vi "HEWH GEA2 Change Mod Sequence.vi"(0 "ComPort":refnum<visa-resource-name>="COM1", 5 "Mode In":T1=enum."StdElectric", 11 "Error In":errorcluster) -> (6 "Mode Set":bool, 15 "Error Out":errorcluster)   [LabVIEW 2009]
uses:
  GEA2/HEWH_Mode.ctl
panel:
  in  "Change Mode Sequence":bool
  in  "Change Mode":bool
  in  "Change Set Point":bool
  in  "Set Point":u8=130
  out "Mode":T1=enum."HighDemand"
  in  "Get Status":bool
  out "Current SetPoint":u8
  in  "OK":bool
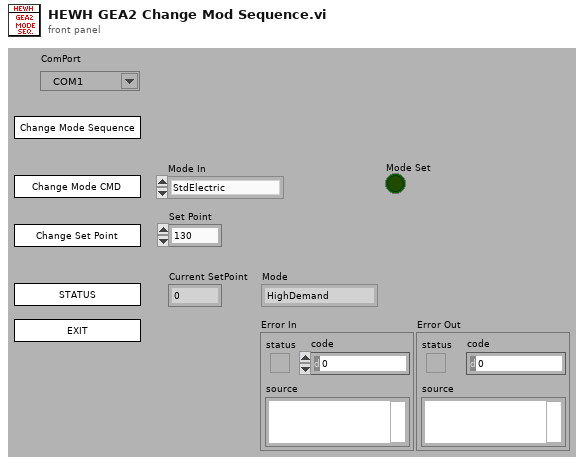
[diagram p1: front panel]
types:
  T1 = typedef "HEWH_Mode.ctl" = enum16{"Hybrid", "StdElectric", "eHeat", "HighDemand", "Unknown"}
  T2 = enum32{"invalid app kind", "Development System", "Run Time System", "Student Edition", "Embedded LabVIEW", "Evaluation", "Custom"}
  T3 = enum32{"Invalid", "Standard", "Closed", "Hidden", "Minimized", "Maximized"}
  T4 = cluster{"Core":cluster{"Current VI Reference":refnum<vi>, "Close Panel on Exit?":bool}, "ComPort":refnum<visa-resource-name>, "Set Point":u8, "Mode In":T1, "Error Status":bool}
  T5 = cluster{"Current VI Reference":refnum<vi>, "Close Panel on Exit?":bool}
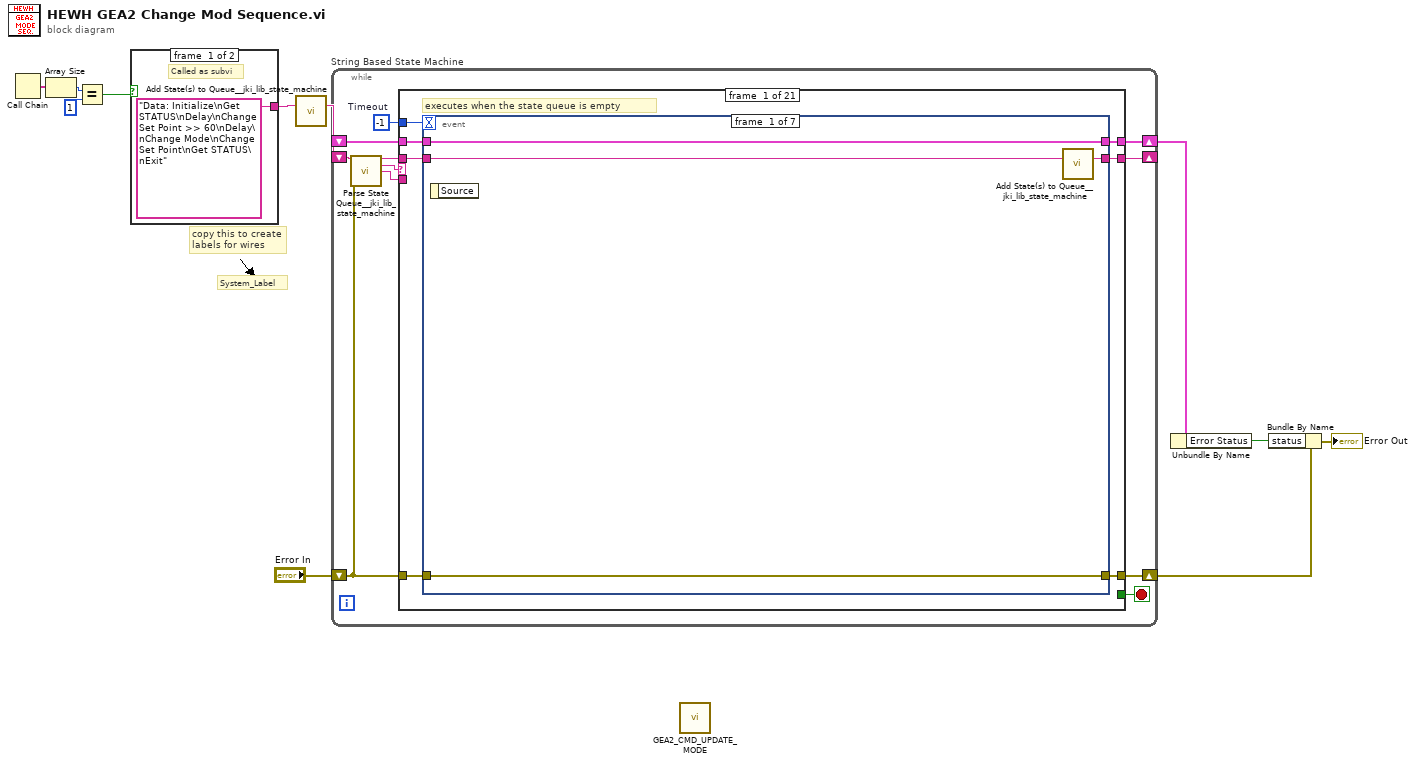
[diagram p0: block diagram]
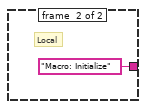
[diagram p2: hidden frame]
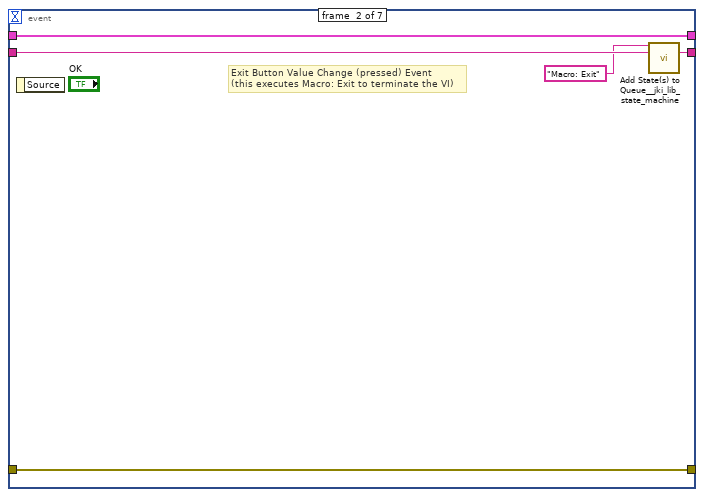
[diagram p3: hidden frame]
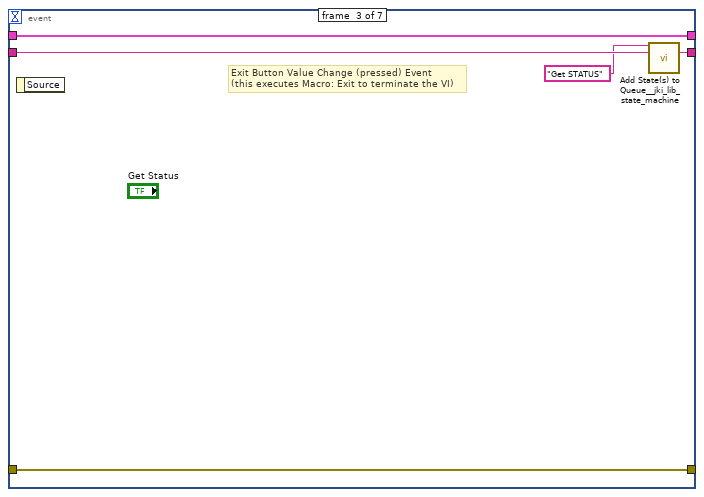
[diagram p4: hidden frame]
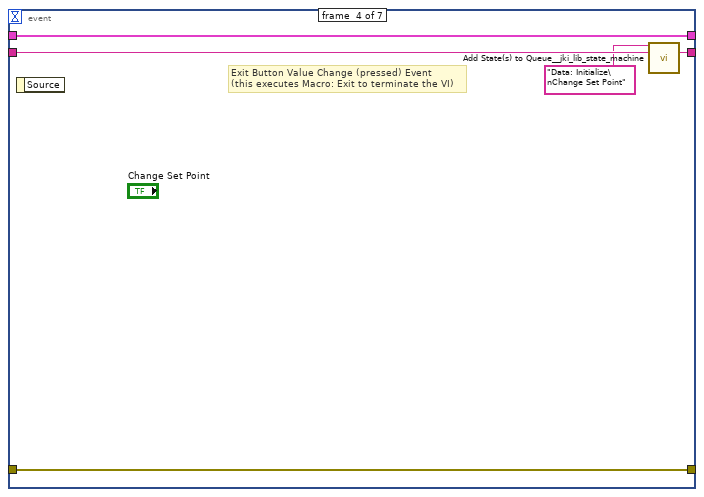
[diagram p5: hidden frame]
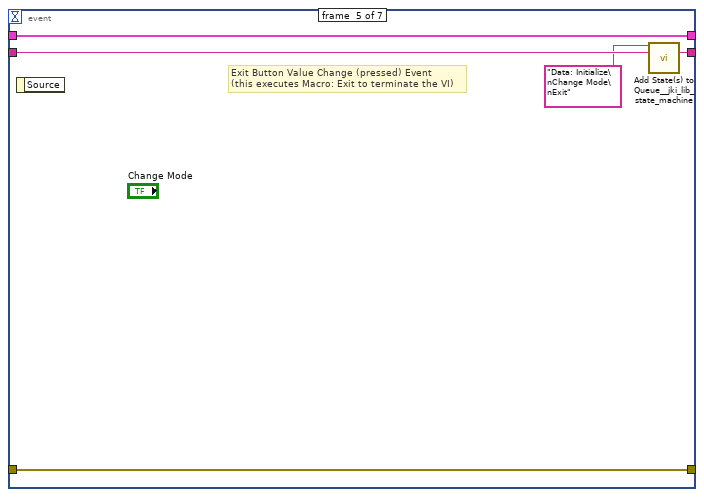
[diagram p6: hidden frame]
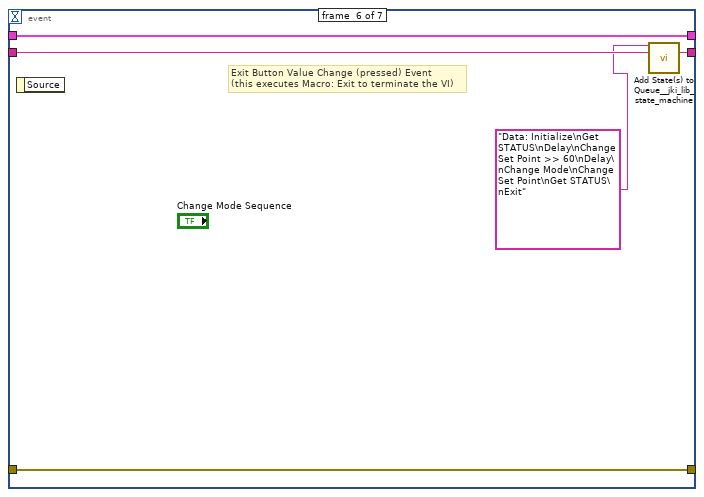
[diagram p7: hidden frame]
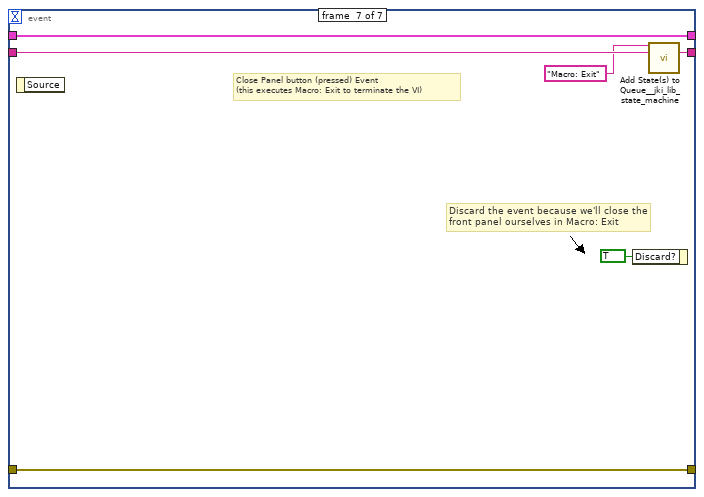
[diagram p8: hidden frame]
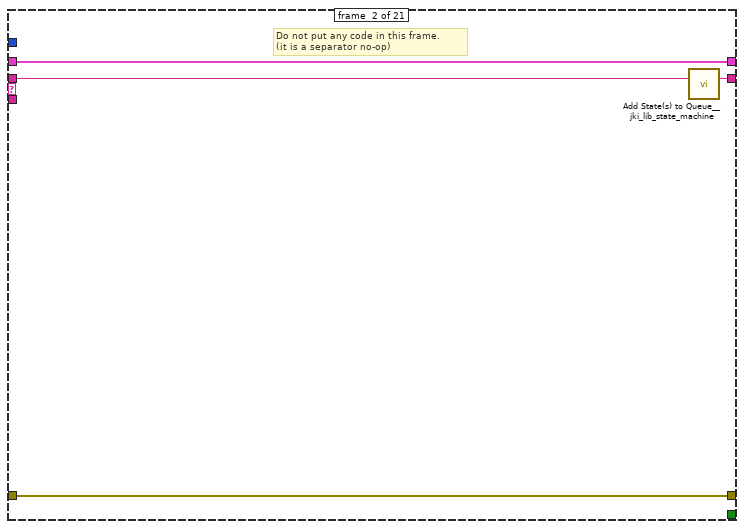
[diagram p9: hidden frame]
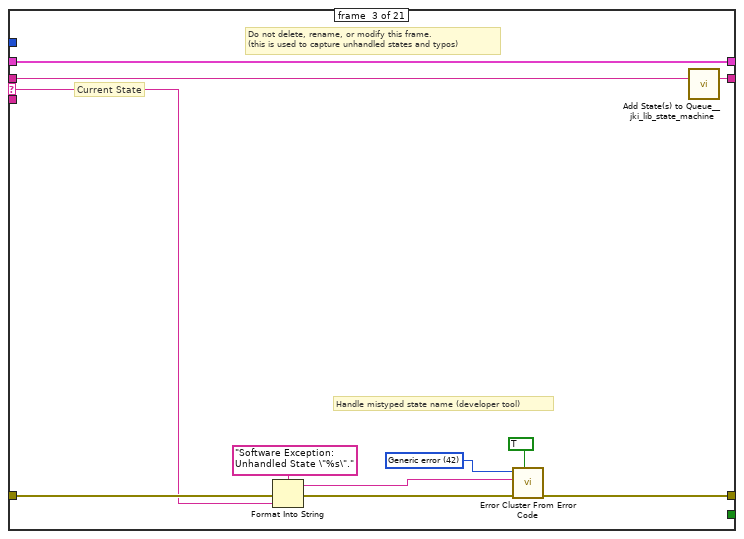
[diagram p10: hidden frame]
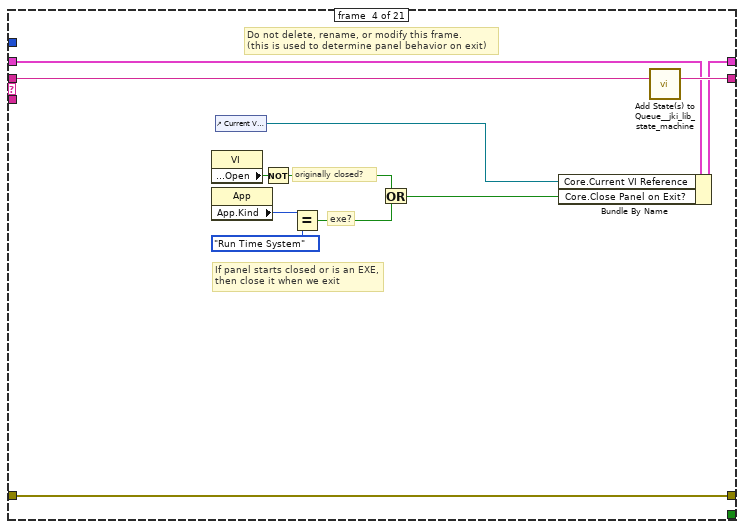
[diagram p11: hidden frame]
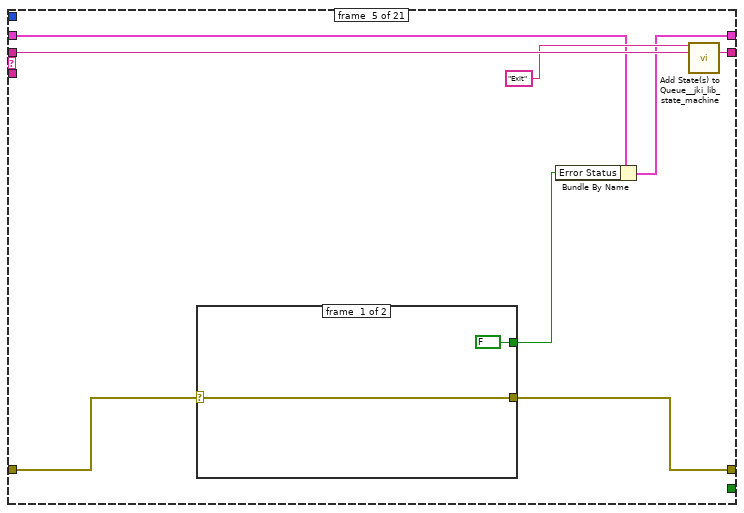
[diagram p12: hidden frame]
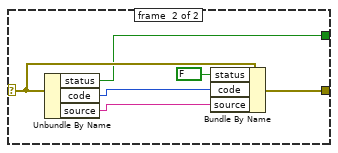
[diagram p13: hidden frame]
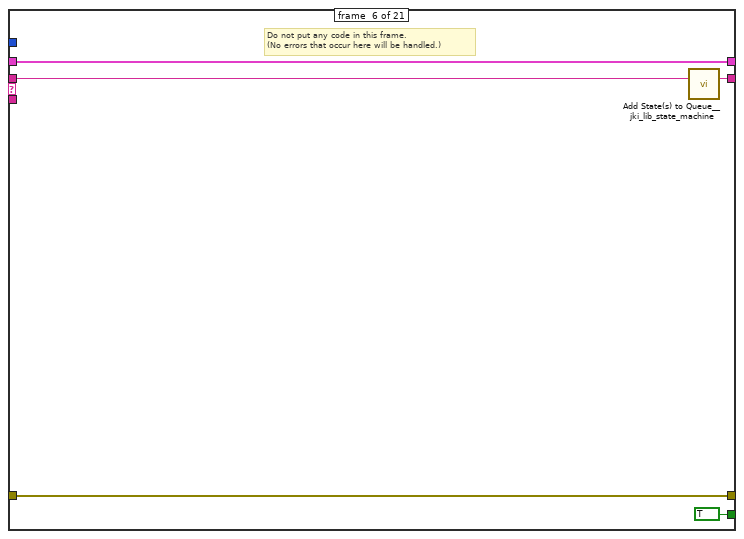
[diagram p14: hidden frame]
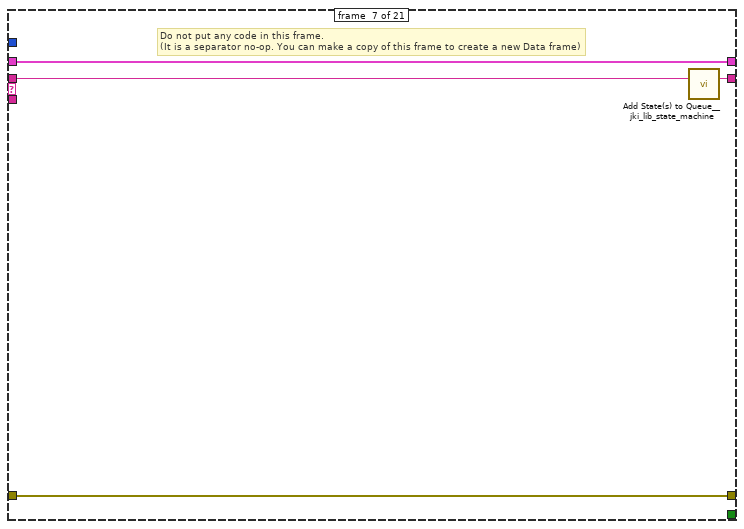
[diagram p15: hidden frame]
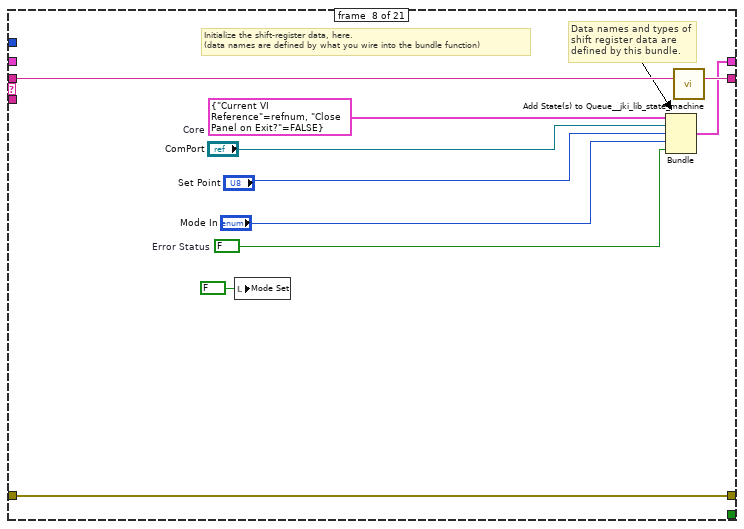
[diagram p16: hidden frame]
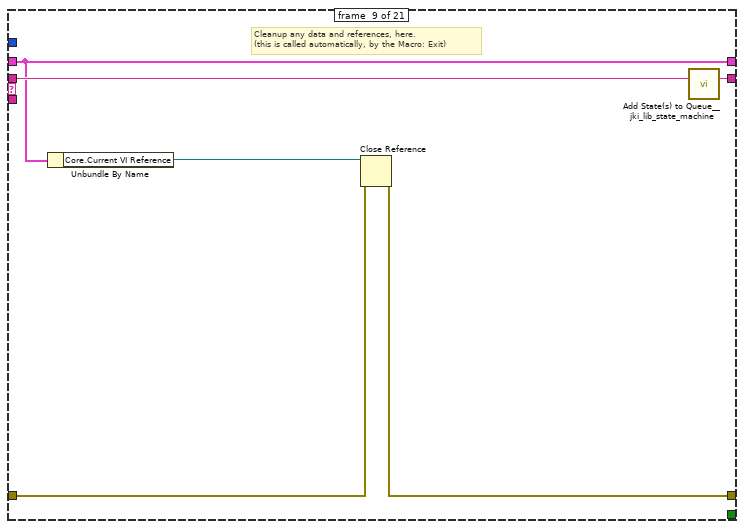
[diagram p17: hidden frame]
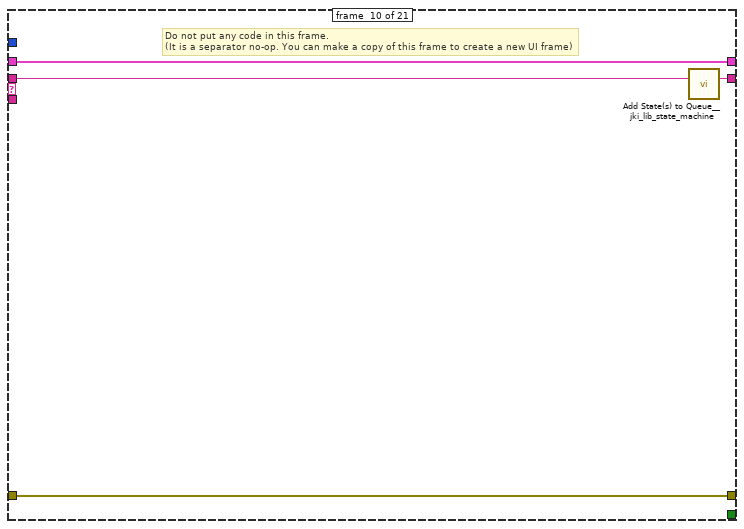
[diagram p18: hidden frame]
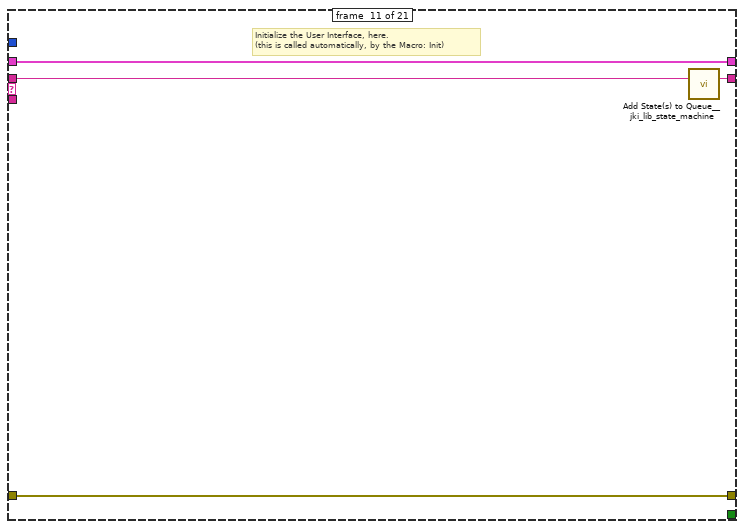
[diagram p19: hidden frame]
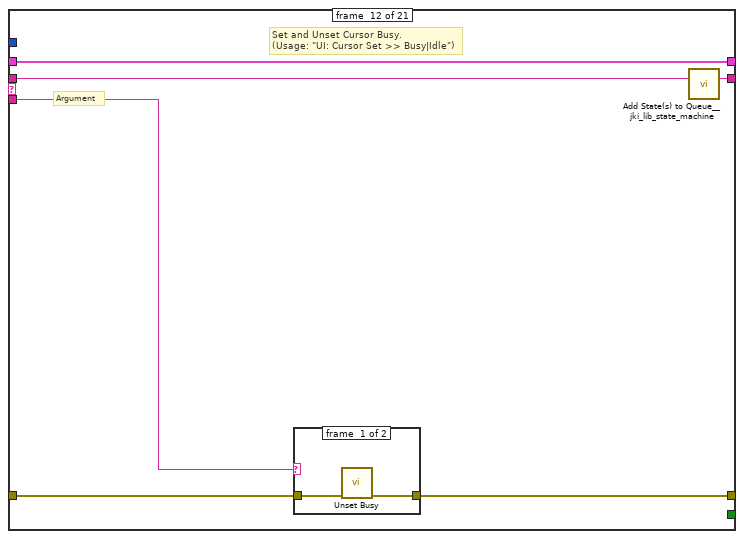
[diagram p20: hidden frame]
diagram:
  # "copy this to create labels for wires"
  # "System_Label"
  n1 = Call Chain() -> (call chain=w7:string[])
  n2 = Array Size(array=w7) -> (size(s)=w8:i32)
  n3 = Equal?(x=w8, y=1) -> (x = y?=w1:bool)
  n4 = case shown="True" w1 {
    tunnel: ["Data: Initialize\nGet STATUS\nDelay\nChange Set Point >> 60\nDelay\nChange Mode\nChange Set Point\nGet STATUS\nExit" "Macro: Initialize"] -> w10
    frame #0 {
      # "Called as subvi"
    }
    frame #1 {
      # "Local"
    }
  }
  n5 = call <vilib>:"Add State(s) to Queue__jki_lib_state_machine.vi"("State(s) in (\"\")"=w10) -> ("States Out"=w11:string)  [unwired: 14 in]
  n6 = while "String Based State Machine" {
    shift-right: [w17] -> w3
    shift-left: _ -> [w16]
    shift-right: [w20] -> w6
    shift-left: "Error In" -> [w14]
    shift-right: [w19] -> _
    shift-left: w11 -> [w21]
    stop <- w18 stop-if-true
    w15 = -1  # Timeout
    n7 = call <vilib>:"Parse State Queue__jki_lib_state_machine.vi"("State Queue"=w21, "Error In (no error)"=w14) -> ("Remaining States"=w23:string, "Current State"=w24:string, "Arguments"=w22:string)  [unwired: 11 in]
    n8 = case shown="\"\", \"Idle\"" w24 {
      selector: w24 -> [_ _ w71 _ _ _ _ _ _ _ _ _ _ _ _ _ _ _ _ _ _]
      tunnel: w23 -> [w31 w70 w75 w93 w101 w114 w118 w128 w134 w138 w142 w148 w159 w185 w190 w200 w204 w218 w231 w246 w254]
      tunnel: w22 -> [_ _ _ _ _ _ _ _ _ _ _ w143 w153 _ _ _ _ _ w223 _ _]
      tunnel: w16 -> [w29 w67 w73 w84 w96 w112 w115 _ w129 w135 w140 w146 w155 w182 w187 w197 w201 w211 w229 w244 w251]
      tunnel: [w28 w68 w77 w90 w97 w111 w116 w125 w130 w136 w139 w144 w156 w183 w188 w198 w202 w214 w226 w241 w250] -> w20
      tunnel: w14 -> [w27 w68 w76 w90 w98 w111 w116 w125 w131 w136 w139 w145 w157 w183 w188 w198 w202 w215 w227 w242 w252]
      tunnel: [w30 w69 w74 w92 w100 w113 w117 w127 w133 w137 w141 w147 w158 w184 w189 w199 w203 w217 w230 w245 w253] -> w19
      tunnel: [_ _ _ _ _ TRUE _ _ _ _ _ _ _ _ _ _ _ _ _ _ _] -> w18
      tunnel: [w26 w67 w73 w91 w95 w112 w115 w126 w129 w135 w140 w146 w155 w182 w187 w197 w201 w210 w229 w244 w251] -> w17
      tunnel: w15 -> [w25 _ _ _ _ _ _ _ _ _ _ _ _ _ _ _ _ _ _ _ _]
      frame #0 {
        # "executes when the state queue is empty"
        n9 = event shown="[4] \"Change Mode\": Value Change" {
          selector: _ -> [_ _ _ _ _ _ _]
          dyn-events: _ -> [_ _ _ _ _ _ _]
          timeout: w25 -> [_ _ _ _ _ _ _]
          tunnel: w31 -> [w35 w40 w45 w50 w55 w60 w66]
          tunnel: [w34 w39 w44 w49 w54 w59 w65] -> w30
          tunnel: w29 -> [w32 w37 w42 w47 w52 w57 w63]
          tunnel: [w33 w38 w43 w48 w53 w58 w64] -> w28
          tunnel: w27 -> [w33 w38 w43 w48 w53 w58 w64]
          tunnel: [w32 w37 w42 w47 w52 w57 w63] -> w26
          event #0 {
            n10 = event-data() -> ()  [unwired: 1 in, 1 out]
            n11 = call <vilib>:"Add State(s) to Queue__jki_lib_state_machine.vi"("State(s) in (\"\")"=w35) -> ("States Out"=w34:string)  [unwired: 14 in]
          }
          event #1 {
            # "Exit Button Value Change (pressed) Event\n(this executes Macro: Exit to terminate the VI)"
            n12 = event-data() -> ()  [unwired: 1 in, 1 out]
            n13 = call <vilib>:"Add State(s) to Queue__jki_lib_state_machine.vi"("State(s) in Front (\"\")"="Macro: Exit", "State(s) in (\"\")"=w40) -> ("States Out"=w39:string)  [unwired: 13 in]
          }
          event #2 {
            # "Exit Button Value Change (pressed) Event\n(this executes Macro: Exit to terminate the VI)"
            n14 = event-data() -> ()  [unwired: 1 in, 1 out]
            n15 = call <vilib>:"Add State(s) to Queue__jki_lib_state_machine.vi"("State(s) in Front (\"\")"="Get STATUS", "State(s) in (\"\")"=w45) -> ("States Out"=w44:string)  [unwired: 13 in]
          }
          event #3 {
            # "Exit Button Value Change (pressed) Event\n(this executes Macro: Exit to terminate the VI)"
            n16 = event-data() -> ()  [unwired: 1 in, 1 out]
            n17 = call <vilib>:"Add State(s) to Queue__jki_lib_state_machine.vi"("State(s) in Front (\"\")"="Data: Initialize\nChange Set Point", "State(s) in (\"\")"=w50) -> ("States Out"=w49:string)  [unwired: 13 in]
          }
          event #4 {
            # "Exit Button Value Change (pressed) Event\n(this executes Macro: Exit to terminate the VI)"
            n18 = event-data() -> ()  [unwired: 1 in, 1 out]
            n19 = call <vilib>:"Add State(s) to Queue__jki_lib_state_machine.vi"("State(s) in Front (\"\")"="Data: Initialize\nChange Mode\nExit", "State(s) in (\"\")"=w55) -> ("States Out"=w54:string)  [unwired: 13 in]
          }
          event #5 {
            # "Exit Button Value Change (pressed) Event\n(this executes Macro: Exit to terminate the VI)"
            n20 = event-data() -> ()  [unwired: 1 in, 1 out]
            n21 = call <vilib>:"Add State(s) to Queue__jki_lib_state_machine.vi"("State(s) in Front (\"\")"="Data: Initialize\nGet STATUS\nDelay\nChange Set Point >> 60\nDelay\nChange Mode\nChange Set Point\nGet STATUS\nExit", "State(s) in (\"\")"=w60) -> ("States Out"=w59:string)  [unwired: 13 in]
          }
          event #6 {
            # "Discard the event because we'll close the front panel ourselves in Macro: Exit"
            # "Close Panel button (pressed) Event\n(this executes Macro: Exit to terminate the VI)"
            n22 = event-data() -> ()  [unwired: 1 in, 1 out]
            n23 = event-data("Discard?"=TRUE) -> ()  [unwired: 1 in, 1 out]
            n24 = call <vilib>:"Add State(s) to Queue__jki_lib_state_machine.vi"("State(s) in Front (\"\")"="Macro: Exit", "State(s) in (\"\")"=w66) -> ("States Out"=w65:string)  [unwired: 13 in]
          }
        }
      }
      frame #1 {
        # "Do not put any code in this frame.\n(it is a separator no-op)"
        n25 = call <vilib>:"Add State(s) to Queue__jki_lib_state_machine.vi"("State(s) in (\"\")"=w70) -> ("States Out"=w69:string)  [unwired: 14 in]
      }
      frame #2 {
        w80 = 42 items=["No error", "Argument error", "Memory is full", "Out of zone", "End of file", "File already open", "Generic file I/O error", "File not found", "File permission error", "Disk is full", "Duplicate path", "Too many files open", "System feature not enabled", "Resource file not found", "Cannot add resource", "Resource not found", "Image not found", "Image memory error", "Pen does not exist", "Config type invalid", "Config token not found", "Config parse error", "Config memory error", "Bad external code format", "Bad external code offset", "External code not present", "Null window", "Destroy window error", "Null menu", "Print aborted", "Bad print record", "Print driver error", "Windows error during printing", "Memory error during printing", "Print dialog error", "Generic print error", "Invalid device refnum", "Device not found", "Device parameter error", "Device unit error", "Cannot open device", "Device call aborted", "Generic error", "Cancelled by user", "Object ID too low", "Object ID too high", "Object not in heap", "Unknown heap", "Unknown object (invalid DefProc)", "Unknown object (DefProc not in table)", "Message out of range", "Invalid (null) method", "Unknown message", "Manager call not supported", "Bad address", "Network operation in progress", "Network operation timed out", "Connection is busy", "Network attribute not supported", "Network error", "Address in use", "System out of memory", "Connection aborted", "Connection refused", "Not connected", "Already connected", "Connection closed", "Initialization error (interapplication manager)", "Bad occurrence", "Wait on unbound occurrence handler", "Occurrence queue overflow", "Datalog type conflict", "Unused", "Unrecognized type (interapplication manager)", "Memory corrupt", "Failed to make temporary DLL", "Old CIN version", "Drag socket not found", "Failed to load drop-object", "Failed to register OLE object", "Failed to release OLE object", "Format specifier type mismatch", "Unknown format specifier", "Too few format specifiers", "Too many format specifiers", "Scan failed", "Newer CIN version", "Error converting to variant", "Runtime menu error", "Password tampered", "Variant attribute not found", "Incompatible variant data type", "Event data is not available", "Event Store is not present", "Occurrence is not found", "Event Queue is not created", "Event info is not available", "Refnum passed is NULL", "Error retrieving Class GUID", "Error retrieving CoClass GUID", "Error retrieving TypeLib GUID.", "Bad built application magic bytes.", "Specific driver is different from the specific driver associated with the Logical Name.", "There is no session opened to the class driver.", "Max Error", "MAX - Error with config objects", "MAX - Error loading configuration", "MAX - Group not supported"]
        # "Current State"
        # "Do not delete, rename, or modify this frame.\n(this is used to capture unhandled states and typos)"
        # "Handle mistyped state name (developer tool)"
        n26 = Format Into String(format string="Software Exception: Unhandled State \"%s\"." ("message"), error in=w76, w71) -> (resulting string=w79:string, error out=w78:errorcluster)  [unwired: 1 in]
        n27 = call <vilib>:"Error Cluster From Error Code.vi"("show call chain? (False)"=TRUE, "error in (no error)"=w78, "error message (\"\")"=w79, "error code (0)"=w80) -> ("error out"=w77:errorcluster)  [unwired: 5 in]
        n28 = call <vilib>:"Add State(s) to Queue__jki_lib_state_machine.vi"("State(s) in (\"\")"=w75) -> ("States Out"=w74:string)  [unwired: 14 in]
      }
      frame #3 {
        # "Do not delete, rename, or modify this frame.\n(this is used to determine panel behavior on exit)"
        # "originally closed?"
        # "exe?"
        # "If panel starts closed or is an EXE, then close it when we exit"
        n29 = property class="VI"() -> ("Front Panel.Open"=w89:bool)  [unwired: 2 in, 2 out]
        n30 = property class="App"() -> ("App.Kind"=w88:T2)  [unwired: 2 in, 2 out]
        n31 = control-ref of="Current VI Reference"() -> (w82:refnum<vi>)
        n32 = Not(x=w89) -> (.not. x?=w86:bool)
        n33 = Equal?(x=w88, y=T2."Run Time System" ("Application:Kind")) -> (x = y?=w85:bool)
        n34 = Or(x=w86, y=w85) -> (x .or. y?=w83:bool)
        n35 = Bundle By Name(cluster=w84, "Core.Current VI Reference"=w82, "Core.Close Panel on Exit?"=w83) -> (w91:T4)
        n36 = call <vilib>:"Add State(s) to Queue__jki_lib_state_machine.vi"("State(s) in (\"\")"=w93) -> ("States Out"=w92:string)  [unwired: 14 in]
      }
      frame #4 {
        n37 = case shown="Error" w98 {
          selector: w98 -> [w103 w109]
          tunnel: [w103 w105] -> w97
          tunnel: [FALSE ("status") w104] -> w94
          frame #0 {
          }
          frame #1 {
            n38 = Unbundle By Name(w109) -> ("status"=w104:bool, "code"=w108:i32, "source"=w107:string)
            n39 = Bundle By Name(cluster=w109, "status"=FALSE, "code"=w108, "source"=w107) -> (w105:errorcluster)
          }
        }
        n40 = Bundle By Name(cluster=w96, "Error Status"=w94) -> (w95:T4)
        n41 = call <vilib>:"Add State(s) to Queue__jki_lib_state_machine.vi"("State(s) in Front (\"\")"="Exit", "State(s) in (\"\")"=w101) -> ("States Out"=w100:string)  [unwired: 13 in]
      }
      frame #5 {
        # "Do not put any code in this frame.\n(No errors that occur here will be handled.)"
        n42 = call <vilib>:"Add State(s) to Queue__jki_lib_state_machine.vi"("State(s) in (\"\")"=w114) -> ("States Out"=w113:string)  [unwired: 14 in]
      }
      frame #6 {
        # "Do not put any code in this frame.\n(It is a separator no-op. You can make a copy of this frame to create a new Data frame)"
        n43 = call <vilib>:"Add State(s) to Queue__jki_lib_state_machine.vi"("State(s) in (\"\")"=w118) -> ("States Out"=w117:string)  [unwired: 14 in]
      }
      frame #7 {
        w120 = FALSE  # Error Status
        w124 = T5 {"Current VI Reference"=refnum, "Close Panel on Exit?"=FALSE}  # Core
        # "Data names and types of shift register data are defined by this bundle."
        # "Initialize the shift-register data, here.\n(data names are defined by what you wire into the bundle function)"
        n44 = local write "Mode Set"(FALSE ("Mode Set")) -> ()
        n45 = Bundle("Core"=w124, "ComPort"="ComPort", "Set Point"="Set Point", "Mode In"="Mode In", "Error Status"=w120) -> (w126:T4)  [unwired: 1 in]
        n46 = call <vilib>:"Add State(s) to Queue__jki_lib_state_machine.vi"("State(s) in (\"\")"=w128) -> ("States Out"=w127:string)  [unwired: 14 in]
      }
      frame #8 {
        # "Cleanup any data and references, here.\n(this is called automatically, by the Macro: Exit)"
        n47 = Unbundle By Name(w129) -> ("Core.Current VI Reference"=w132:refnum<vi>)
        n48 = Close Reference(reference=w132, error in (no error)=w131) -> (error out=w130:errorcluster)
        n49 = call <vilib>:"Add State(s) to Queue__jki_lib_state_machine.vi"("State(s) in (\"\")"=w134) -> ("States Out"=w133:string)  [unwired: 14 in]
      }
      frame #9 {
        # "Do not put any code in this frame.\n(It is a separator no-op. You can make a copy of this frame to create a new UI frame)"
        n50 = call <vilib>:"Add State(s) to Queue__jki_lib_state_machine.vi"("State(s) in (\"\")"=w138) -> ("States Out"=w137:string)  [unwired: 14 in]
      }
      frame #10 {
        # "Initialize the User Interface, here.\n(this is called automatically, by the Macro: Init)"
        n51 = call <vilib>:"Add State(s) to Queue__jki_lib_state_machine.vi"("State(s) in (\"\")"=w142) -> ("States Out"=w141:string)  [unwired: 14 in]
      }
      frame #11 {
        # "Argument"
        # "Set and Unset Cursor Busy.\n(Usage: \"UI: Cursor Set >> Busy|Idle\")"
        n52 = case shown="\"Idle\", Default" w143 {
          tunnel: w145 -> [w150 w152]
          tunnel: [w149 w151] -> w144
          frame #0 {
            n53 = call <vilib>:"Unset Busy.vi"("error in (no error)"=w150) -> ("error out"=w149:errorcluster)  [unwired: 10 in]
          }
          frame #1 {
            n54 = call <vilib>:"Set Busy.vi"("error in (no error)"=w152) -> ("error out"=w151:errorcluster)  [unwired: 9 in, 1 out]
          }
        }
        n55 = call <vilib>:"Add State(s) to Queue__jki_lib_state_machine.vi"("State(s) in (\"\")"=w148) -> ("States Out"=w147:string)  [unwired: 14 in]
      }
      frame #12 {
        # "Argument"
        # "Set Front Panel Open or Closed\n(Usage: \"UI: Front Panel State >> Open|Close\")"
        n56 = Unbundle By Name(w155) -> ("Core.Current VI Reference"=w154:refnum<vi>)
        n57 = case shown="\"Open\", Default" w153 {
          tunnel: w157 -> [w163 w176]
          tunnel: [w165 w177] -> w156
          tunnel: w154 -> [w164 w174]
          frame #0 {
            n58 = property class="VI"(reference=w164, error in=w163) -> (reference out=w161:refnum<vi>, error out=w162:errorcluster, "Front Panel.Open"=w160:bool)
            n59 = case shown="False" w160 {
              tunnel: [w168 w171] -> w165
              tunnel: w162 -> [w167 w171]
              tunnel: w161 -> [w166 _]
              frame #0 {
                n60 = invoke class="VI" method="FP.Open"(reference=w166, error in=w167, "Activate"=TRUE, "State"=T3."Standard") -> (error out=w168:errorcluster)  [unwired: 1 in, 4 out]
              }
              frame #1 {
              }
            }
          }
          frame #1 {
            n61 = property class="VI"(reference=w174, error in=w176) -> (reference out=w173:refnum<vi>, error out=w175:errorcluster, "Front Panel.Open"=w172:bool)
            n62 = case shown="True" w172 {
              tunnel: [w178 w181] -> w177
              tunnel: w175 -> [w178 w180]
              tunnel: w173 -> [_ w179]
              frame #0 {
              }
              frame #1 {
                n63 = invoke class="VI" method="FP.Close"(reference=w179, error in=w180) -> (error out=w181:errorcluster)  [unwired: 1 in, 2 out]
              }
            }
          }
        }
        n64 = call <vilib>:"Add State(s) to Queue__jki_lib_state_machine.vi"("State(s) in (\"\")"=w159) -> ("States Out"=w158:string)  [unwired: 14 in]
      }
      frame #13 {
        # "Do not put any code in this frame.\n(It is a separator no-op. You can make a copy of this frame to create a new Macro frame)"
        n65 = call <vilib>:"Add State(s) to Queue__jki_lib_state_machine.vi"("State(s) in (\"\")"=w185) -> ("States Out"=w184:string)  [unwired: 14 in]
      }
      frame #14 {
        w186 = "Data: Initialize\nInitialize Core Data\nUI: Initialize\nUI: Front Panel State >> Open"  # Data: Initialize Initialize Core Data UI: Initialize UI: Front Panel State >> Open
        # "Initialization Macro\n(This is called once, when the VI starts)"
        n66 = call <vilib>:"Add State(s) to Queue__jki_lib_state_machine.vi"("State(s) in Front (\"\")"=w186, "State(s) in (\"\")"=w190) -> ("States Out"=w189:string)  [unwired: 13 in]
      }
      frame #15 {
        # "Exit Macro\n(This is called once, when the VI exits)"
        n67 = Unbundle By Name(w197) -> ("Core.Close Panel on Exit?"=w196:bool)
        n68 = Select(t="UI: Front Panel State >> Close", s=w196, f="") -> (s? t:f=w193:string)
        n69 = call <vilib>:"Add State(s) to Queue__jki_lib_state_machine.vi"("State(s) in (\"\")"=w193, "State(s) at Back (\"\")"="Data: Cleanup\nExit") -> ("States Out"=w191:string)  [unwired: 13 in]
        n70 = call <vilib>:"Add State(s) to Queue__jki_lib_state_machine.vi"("State(s) in Front (\"\")"=w191, "State(s) in (\"\")"=w200) -> ("States Out"=w199:string)  [unwired: 13 in]
      }
      frame #16 {
        # "Template Separator\n(You can make a copy of, or modify, this frame)"
        n71 = call <vilib>:"Add State(s) to Queue__jki_lib_state_machine.vi"("State(s) in (\"\")"=w204) -> ("States Out"=w203:string)  [unwired: 14 in]
      }
      frame #17 {
        # "Your code here.\n(You can make a copy of, or modify, this frame)"
        n72 = Unbundle By Name(w211) -> ("Mode In"=w205:T1, "ComPort"=w216:refnum<visa-resource-name>)
        n73 = call "GEA2_RQST_STATUS_QUERY.vi"("ComPort"=w216, "Error In"=w215) -> ("ACK"=w213:bool, "Mode"=w206:T1, "Current SetPoint"=w209:u8, "Error Out"=w214:errorcluster)  [unwired: 9 in, 1 out]
        "Current SetPoint" <- w209
        "Mode" <- w206
        n74 = Equal?(x=w205, y=w206) -> (x = y?=w207:bool)
        "Mode Set" <- w207
        n75 = Or(x=w207, y=w213) -> (x .or. y?=w208:bool)
        n76 = Bundle By Name(cluster=w211, "Set Point"=w209) -> (w210:T4)
        n77 = case shown="False" w208 {
          tunnel: ["Finish" ("State(s) in Front (\"\")") "" ("State(s) in Front (\"\")")] -> w212
          frame #0 {
          }
          frame #1 {
          }
        }
        n78 = call <vilib>:"Add State(s) to Queue__jki_lib_state_machine.vi"("State(s) in Front (\"\")"=w212, "State(s) in (\"\")"=w218) -> ("States Out"=w217:string)  [unwired: 13 in]
      }
      frame #18 {
        # "Set Front Panel Open or Closed\n(Usage: \"UI: Front Panel State >> xx)\nIf set point left blank, use input control"
        n79 = Unbundle By Name(w229) -> ("ComPort"=w228:refnum<visa-resource-name>, "Set Point"=w221:u8)
        n80 = case shown="\"60\", Default" w223 {
          selector: w223 -> [_ w235]
          tunnel: [w232 w233] -> w222
          tunnel: w221 -> [w232 _]
          frame #0 {
          }
          frame #1 {
            n81 = Decimal String To Number(string=w235) -> (number=w234:i32)  [unwired: 2 in, 1 out]
            n82 = To Unsigned Byte Integer(number=w234) -> (unsigned 8bit integer=w233:u8)
          }
        }
        n83 = call "GEA2_CMD_WRITE_SETPOINTS.vi"("ComPort"=w228, "Set Point"=w222, "Error In"=w227) -> ("ACK"=w225:bool, "Error Out"=w226:errorcluster)  [unwired: 11 in]
        n84 = case shown="False" w225 {
          tunnel: ["Finish" ("State(s) in Front (\"\")") "" ("State(s) in Front (\"\")")] -> w224
          frame #0 {
          }
          frame #1 {
          }
        }
        n85 = call <vilib>:"Add State(s) to Queue__jki_lib_state_machine.vi"("State(s) in Front (\"\")"=w224, "State(s) in (\"\")"=w231) -> ("States Out"=w230:string)  [unwired: 13 in]
      }
      frame #19 {
        # "Set Front Panel Open or Closed\n(Usage: \"UI: Front Panel State >> xx)\nIf set point left blank, use input control"
        n86 = Unbundle By Name(w244) -> ("ComPort"=w243:refnum<visa-resource-name>, "Mode In"=w238:T1)
        n87 = call "GEA2_CMD_UPDATE_MODE.vi"("ComPort"=w243, "Mode"=w238, "Error In"=w242) -> ("ACK"=w240:bool, "Error Out"=w241:errorcluster)  [unwired: 10 in, 1 out]
        n88 = case shown="True" w240 {
          tunnel: ["Finish" ("State(s) in Front (\"\")") "" ("State(s) in Front (\"\")")] -> w239
          frame #0 {
          }
          frame #1 {
          }
        }
        n89 = call <vilib>:"Add State(s) to Queue__jki_lib_state_machine.vi"("State(s) in Front (\"\")"=w239, "State(s) in (\"\")"=w246) -> ("States Out"=w245:string)  [unwired: 13 in]
      }
      frame #20 {
        # "Delay needs to be > 1 second"
        n90 = call "Delay mS.vi"("Error In"=w252, "milliseconds to wait"=u32 2000) -> ("Error Out"=w250:errorcluster)  [unwired: 13 in]
        n91 = call <vilib>:"Add State(s) to Queue__jki_lib_state_machine.vi"("State(s) in (\"\")"=w254) -> ("States Out"=w253:string)  [unwired: 14 in]
      }
    }
  }
  n92 = call "GEA2_CMD_UPDATE_MODE.vi"() -> ()  [unwired: 13 in, 3 out]
  n93 = Unbundle By Name(w3) -> ("Error Status"=w2:bool)
  n94 = Bundle By Name(cluster=w6, "status"=w2) -> (→"Error Out":errorcluster)
